vi "Heat Equation (Simplified Finite Difference).vi"() -> ()   [LabVIEW 2023]
doc: "Calculates the heating process of a metal plate based on the dimensions, boundary conditions, and initial temperature of the plate."
panel:
  in  "starting temperature":sgl=5.0 format="%0.2f"
  in  "Stop":bool
  in  "top temp":sgl(slide)=50.847458 scale=0.0..100.0
  in  "right temp":sgl(slide)=77.55102 scale=0.0..100.0
  in  "bottom temp":sgl(slide)=20.338984 scale=0.0..100.0
  in  "left temp":sgl(slide)=41.836735 scale=0.0..100.0
  in  "width y":i32=100 min=1 max=1000
  in  "width x":i32=150 min=1 max=1000
  out "Solution":sgl[][](graph)
  # "Overview: Demonstrates heat conduction on a metal plate.\nRequirements: LabVIEW Full Development System\nInstructions: \n1. Set the desired width x, width y, and starting temperature and run the VI.\n2. Change the boundary (left, right, top, bottom) temperatures and observe the simulated heat propagation on a metal plate.\n3. Click Stop to stop the VI."
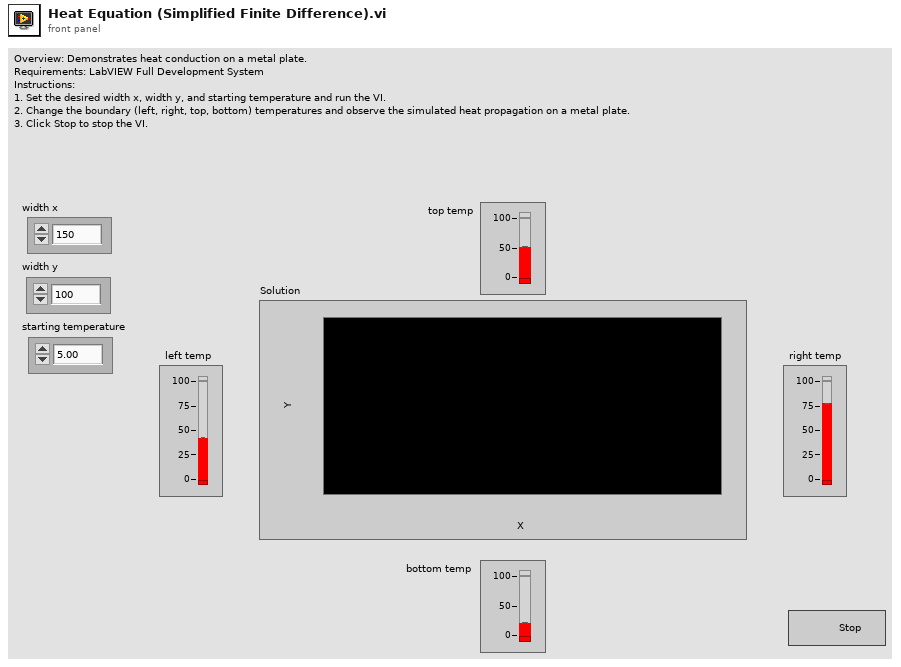
[diagram p1: front panel]
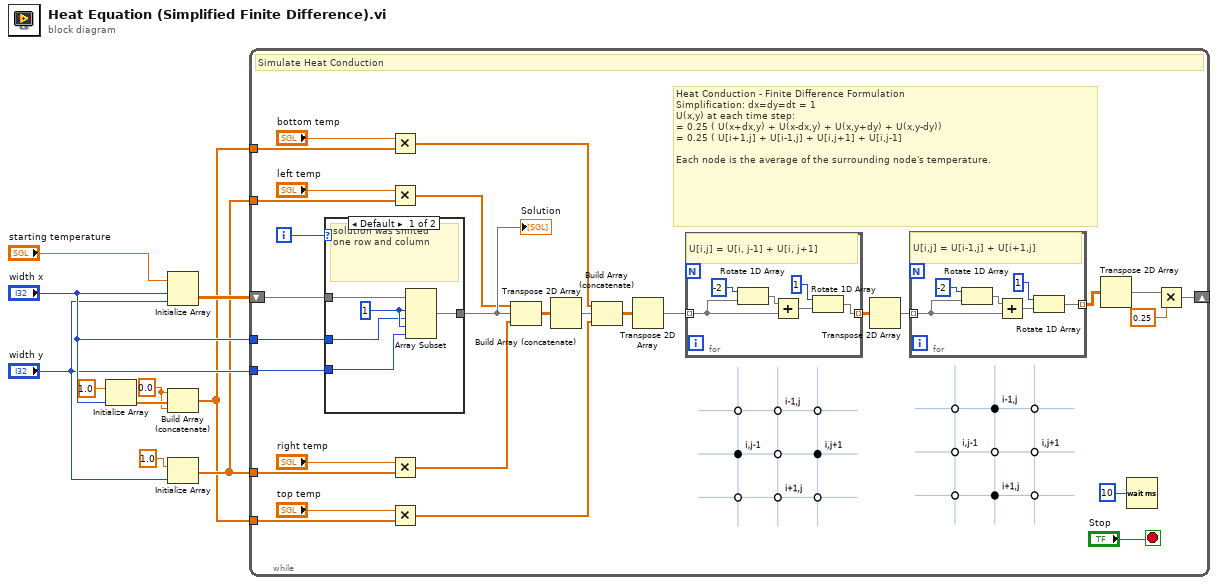
[diagram p0: block diagram]
diagram:
  w7 = sgl 0.0
  n1 = Initialize Array(sgl 1.0 ("element"), "width x") -> (w8:sgl[])
  n2 = Initialize Array("starting temperature", "width x", "width y") -> (w9:sgl[][])
  n3 = Build Array (concatenate)(w7, w8, w7) -> (w1:sgl[])
  n4 = Initialize Array(sgl 1.0 ("element"), "width y") -> (w2:sgl[])
  n5 = while {
    tunnel: "width y" -> [w36]
    tunnel: "width x" -> [w37]
    shift-left: w9 -> [w33]
    shift-right: [w30] -> _
    tunnel: w1 -> [w14]
    tunnel: w2 -> [w18]
    tunnel: w2 -> [w12]
    tunnel: w1 -> [w11]
    i -> [w13]
    stop <- "Stop" stop-if-true
    # "Heat Conduction - Finite Difference Formulation\nSimplification: dx=dy=dt = 1\nU(x,y) at each time step:\n= 0.25 ( U(x+dx,y) + U(x-dx,y) + U(x,y+dy) + U(x,y-dy))\n= 0.25 ( U[i+1,j] + U[i-1,j] + U[i,j+1] + U[i,j-1]\n\nEach node is the average of the surrounding node's temperature."
    # "Simulate Heat Conduction"
    n6 = case shown="Default" w13 {
      tunnel: [w46 w51] -> w24
      tunnel: w33 -> [w50 w51]
      tunnel: w37 -> [w48 _]
      tunnel: w36 -> [w47 _]
      frame Default {
        w49 = 1
        # "solution was shifted\none row and column"
        n7 = Array Subset(array=w50, index (row)=w49, length (row)=w48, index (col)=w49, length (col)=w47) -> (w46:sgl[][])
      }
      frame 0 {
      }
    }
    "Solution" <- w24
    n8 = Multiply(x="bottom temp", y=w11) -> (x*y=w20:sgl[])
    n9 = Multiply(x="left temp", y=w12) -> (x*y=w17:sgl[])
    n10 = Multiply(x="right temp", y=w18) -> (x*y=w19:sgl[])
    n11 = Multiply(x="top temp", y=w14) -> (x*y=w22:sgl[])
    n12 = Build Array (concatenate)(w17, w24, w19) -> (w39:sgl[][])
    n13 = Transpose 2D Array(2D array=w39) -> (transposed array=w38:sgl[][])
    n14 = Build Array (concatenate)(w20, w38, w22) -> (w35:sgl[][])
    n15 = Transpose 2D Array(2D array=w35) -> (transposed array=w34:sgl[][])
    n16 = for {
      tunnel: w34 -> [w56] mode=indexing
      tunnel: [w52] -> w28 mode=indexing
      # "U[i,j] = U[i, j-1] + U[i, j+1]"
      n17 = Rotate 1D Array(1:w56, 2:-2) -> (0:w53:sgl[])
      n18 = Add(x=w53, y=w56) -> (x+y=w55:sgl[])
      n19 = Rotate 1D Array(1:w55, 2:1) -> (0:w52:sgl[])
    }
    n20 = Transpose 2D Array(2D array=w28) -> (transposed array=w27:sgl[][])
    n21 = for {
      tunnel: w27 -> [w44] mode=indexing
      tunnel: [w40] -> w26 mode=indexing
      # "U[i,j] = U[i-1,j] + U[i+1,j]"
      n22 = Rotate 1D Array(1:w44, 2:-2) -> (0:w41:sgl[])
      n23 = Add(x=w41, y=w44) -> (x+y=w43:sgl[])
      n24 = Rotate 1D Array(1:w43, 2:1) -> (0:w40:sgl[])
    }
    n25 = Transpose 2D Array(2D array=w26) -> (transposed array=w32:sgl[][])
    n26 = Wait (ms)(milliseconds to wait=u32 10) -> ()  [unwired: 1 out]
    n27 = Multiply(x=w32, y=sgl 0.25) -> (x*y=w30:sgl[][])
  }
